vi "Apply.vi"(8 "error in":errorcluster, 11 "Thermometer DAQmx RTD Cont CFG in":refnum<class "Thermometer DAQmx RTD Cont CFG.lvclass">) -> (0 "error out":errorcluster, 3 "Thermometer DAQmx RTD Cont CFG out":refnum<class "Thermometer DAQmx RTD Cont CFG.lvclass">)   [LabVIEW 2023, in "DAQmx Simulated CFGs.lvlib" / "Thermometer DAQmx RTD Cont CFG.lvclass"]
uses:
  Thermometer DAQmx RTD Cont CFG.lvclass
  Configuration/Configuration JSON/Configuration JSON Base/CFG JSON.lvclass
  Thermometer DAQmx RTD Cont CFG/Thermometer DAQmx RTD Cont CFG.lvclass
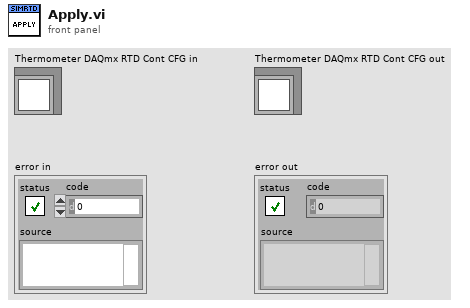
[diagram p1: front panel]
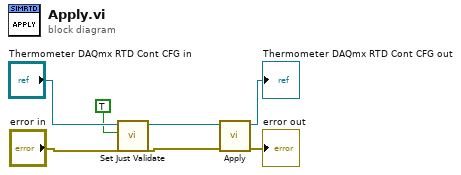
[diagram p0: block diagram]
diagram:
  n1 = call "Set Just Validate.vi"("Just Validate"=TRUE, "CFG JSON Base in"="Thermometer DAQmx RTD Cont CFG in") -> ("CFG JSON Base out"=w3:refnum<class "Thermometer DAQmx RTD Cont CFG.lvclass">)  [unwired: 9 in]
  n2 = call-parent "Apply.vi"("error in"="error in", "Thermometer DAQmx RTD Cont CFG in"=w3) -> ("error out"=→"error out":errorcluster, "Thermometer DAQmx RTD Cont CFG out"=→"Thermometer DAQmx RTD Cont CFG out":refnum<class "Thermometer DAQmx RTD Cont CFG.lvclass">)  [unwired: 8 in]
